vi "Find Devices of Specified Type.vi"(8 "error in (no error)":errorcluster, 9 "Function Name":string, 10 "Hardware Type":string, 11 "Controller in":refnum<class "Controller.lvclass">) -> (0 "error out":errorcluster, 3 "Controller out":refnum<class "Controller.lvclass">)   [LabVIEW 2016, in "Controller Actor.lvlib" / "Controller.lvclass"]
uses:
  <userlib>/Common Components/Controller/Controller.lvclass
  C:/Program Files (x86)/National Instruments/LabVIEW 2016/vi.lib/ActorFramework/Actor/Actor.lvclass
  <vilib>/ActorFramework/Actor/Actor.lvclass/Actor.ctl
  <vilib>/ActorFramework/Message Enqueuer/Message Enqueuer.lvclass/Message Enqueuer.ctl
  <userlib>/Common Components/Controller/Messages/Respond with Devices for Function Msg/Respond with Devices for Function Msg.lvclass/Respond with Devices for Function Msg.ctl
  <vilib>/ActorFramework/Message Enqueuer/Init from Existing Queue.vi
  <vilib>/ActorFramework/Message Enqueuer/Enqueue.vi
  <userlib>/Common Components/Controller/Messages/Respond with Devices for Function Msg/Respond with Devices for Function Msg.lvclass
  C:/Program Files (x86)/National Instruments/LabVIEW 2016/vi.lib/ActorFramework/Message/Message.lvclass
  <vilib>/ActorFramework/Message Priority Queue/Priority Enqueue.vi
  <vilib>/ActorFramework/Message Enqueuer/Message Enqueuer.lvclass
  <vilib>/ActorFramework/Actor/Actor.lvclass
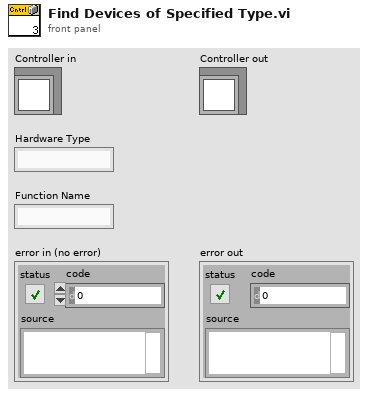
[diagram p1: front panel]
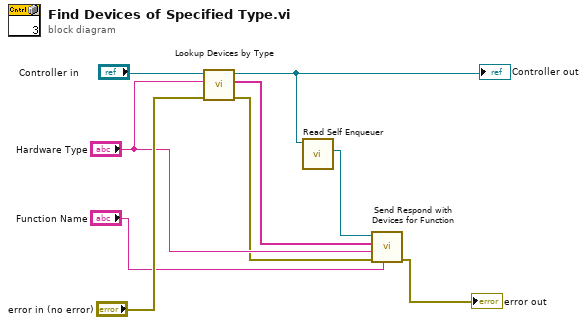
[diagram p0: block diagram]
diagram:
  n1 = call <userlib>:"Lookup Devices by Type.vi"("error in (no error)"="error in (no error)", "Hardware Type"="Hardware Type", "Controller in"="Controller in") -> ("error out"=w2:errorcluster, "Matching Devices"=w5:string[], "Controller out"=w7:refnum<class "Controller.lvclass">)  [unwired: 6 in]
  "Controller out" <- w7
  n2 = call <vilib>:"Read Self Enqueuer.vi"("Actor"=w7) -> ("Self Enqueuer"=w6:refnum<class "Message Enqueuer.lvclass">)  [unwired: 10 in]
  n3 = call <userlib>:"Send Respond with Devices for Function.vi"("Function Name"="Function Name", "error in (no error)"=w2, "Hardware Type"="Hardware Type", "Matching Devices"=w5, "Message Enqueuer"=w6) -> ("error out"=→"error out":errorcluster)  [unwired: 5 in, 1 out]
